vi "Problemas de monitoreo.vi"() -> ()   [LabVIEW 2020]
uses:
  <vilib>/Instr/_visa.llb/VISA Configure Serial Port (Instr).vi
panel:
  out "concatenated string 2":string
  in  "string":string
  in  "Boolean 2":bool
  in  "stop":bool
  in  "Boolean":bool
  out "concatenated string":string
  in  "VISA resource name":refnum<visa-resource-name>
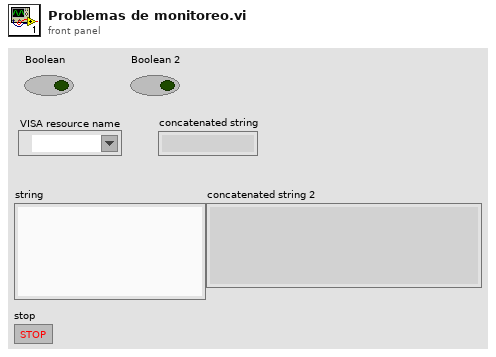
[diagram p1: front panel]
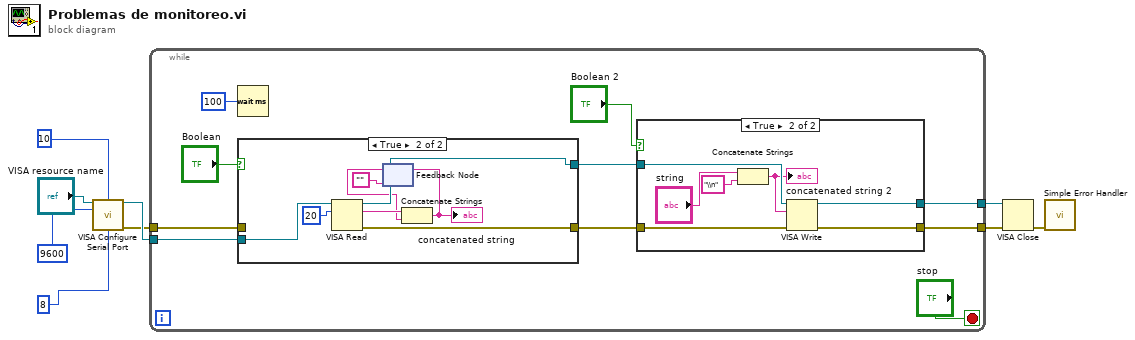
[diagram p0: block diagram]
diagram:
  n1 = call-poly "VISA Configure Serial Port"("VISA resource name"="VISA resource name", "termination char\n(0xA = '\\n' = LF)"=u8 10 ("termination char\n(0xA = '\\n' = LF)"), "baud rate (9600)"=u32 9600, "data bits (8)"=u16 8) -> ("VISA resource name out"=w6:refnum<visa-resource-name>, "error out"=w5:errorcluster)  [unwired: 10 in]
  n2 = while {
    tunnel: w6 -> [w18]
    tunnel: w5 -> [w14]
    tunnel: [w11] -> w4
    tunnel: [w10] -> w3
    stop <- "stop" stop-if-true
    n3 = Wait (ms)(milliseconds to wait=u32 100) -> ()  [unwired: 1 out]
    n4 = case shown="True" "Boolean" {
      tunnel: w18 -> [w30 w36]
      tunnel: [w30 w35] -> w17
      tunnel: w14 -> [w29 _]
      tunnel: [w29 w34] -> w13
      frame False {
      }
      frame True {
        n5 = VISA Read(VISA resource name=w36, byte count=u32 20) -> (VISA resource name out=w35:refnum<visa-resource-name>, read buffer=w37:string, error out=w34:errorcluster)  [unwired: 1 in, 1 out]
        n6 = feedback #1("") -> (w32:string)
        n7 = Concatenate Strings(w37, w32) -> (w33:string)
        "concatenated string" <- w33
        n8 = feedback-in #1(w33) -> ()
      }
    }
    n9 = case shown="True" "Boolean 2" {
      tunnel: w17 -> [w20 w27]
      tunnel: w13 -> [w21 w25]
      tunnel: [w20 w28] -> w10
      tunnel: [w21 w26] -> w11
      frame False {
      }
      frame True {
        n10 = Concatenate Strings("string", "\\n" ("string")) -> (w24:string)
        "concatenated string 2" <- w24
        n11 = VISA Write(VISA resource name=w27, write buffer=w24, error in (no error)=w25) -> (VISA resource name out=w28:refnum<visa-resource-name>, error out=w26:errorcluster)  [unwired: 1 out]
      }
    }
  }
  n12 = VISA Close(VISA resource name=w3, error in (no error)=w4) -> (error out=w2:errorcluster)
  n13 = call <vilib>:"Simple Error Handler.vi"("error in (no error)"=w2) -> ()  [unwired: 4 in, 5 out]
